vi "Common_UpdateAttributes.vi"(1 "ClassPath/LvClassRef":variant, 2 "NewAttributes":string, 3 "ClassInfo":T4[](array[typedef]), 5 "error in (no error)":errorcluster, 6 "Don't Prompt (False)":bool, 7 "Attributes":T1[](array[typedef]), 8 "Stereotype":string, 9 "Ctl-Description":string) -> (15 "CtlPath":path, 18 "Cancel":bool=TRUE, 19 "error out":errorcluster)   [LabVIEW 2020]
uses:
  <resource>/Framework/Providers/Open_GDS/ClassProviders/Common/CommonVIs/CommonVIs_ClassNamePathType.ctl
  <resource>/Framework/Providers/Open_GDS/ClassProviders/Common/CommonVIs/CommonVIs_AttributeType.ctl
  <resource>/Framework/Providers/Open_GDS/ClassProviders/Common/CommonVIs/CommonVIs_AttributeDataType.ctl
  <resource>/Framework/Providers/Open_GDS/ClassProviders/Common/String/GDSString_AccessScopeModifierType.ctl
  <resource>/Framework/Providers/Open_GDS/ClassProviders/Provider_BaseClassInterface/ClassReader_class/ClassReader.lvclass
panel:
  out "Path":path
  in  "Backup":bool
  out "New Attributes":string
  in  "Cancel":bool
  in  "OK":bool
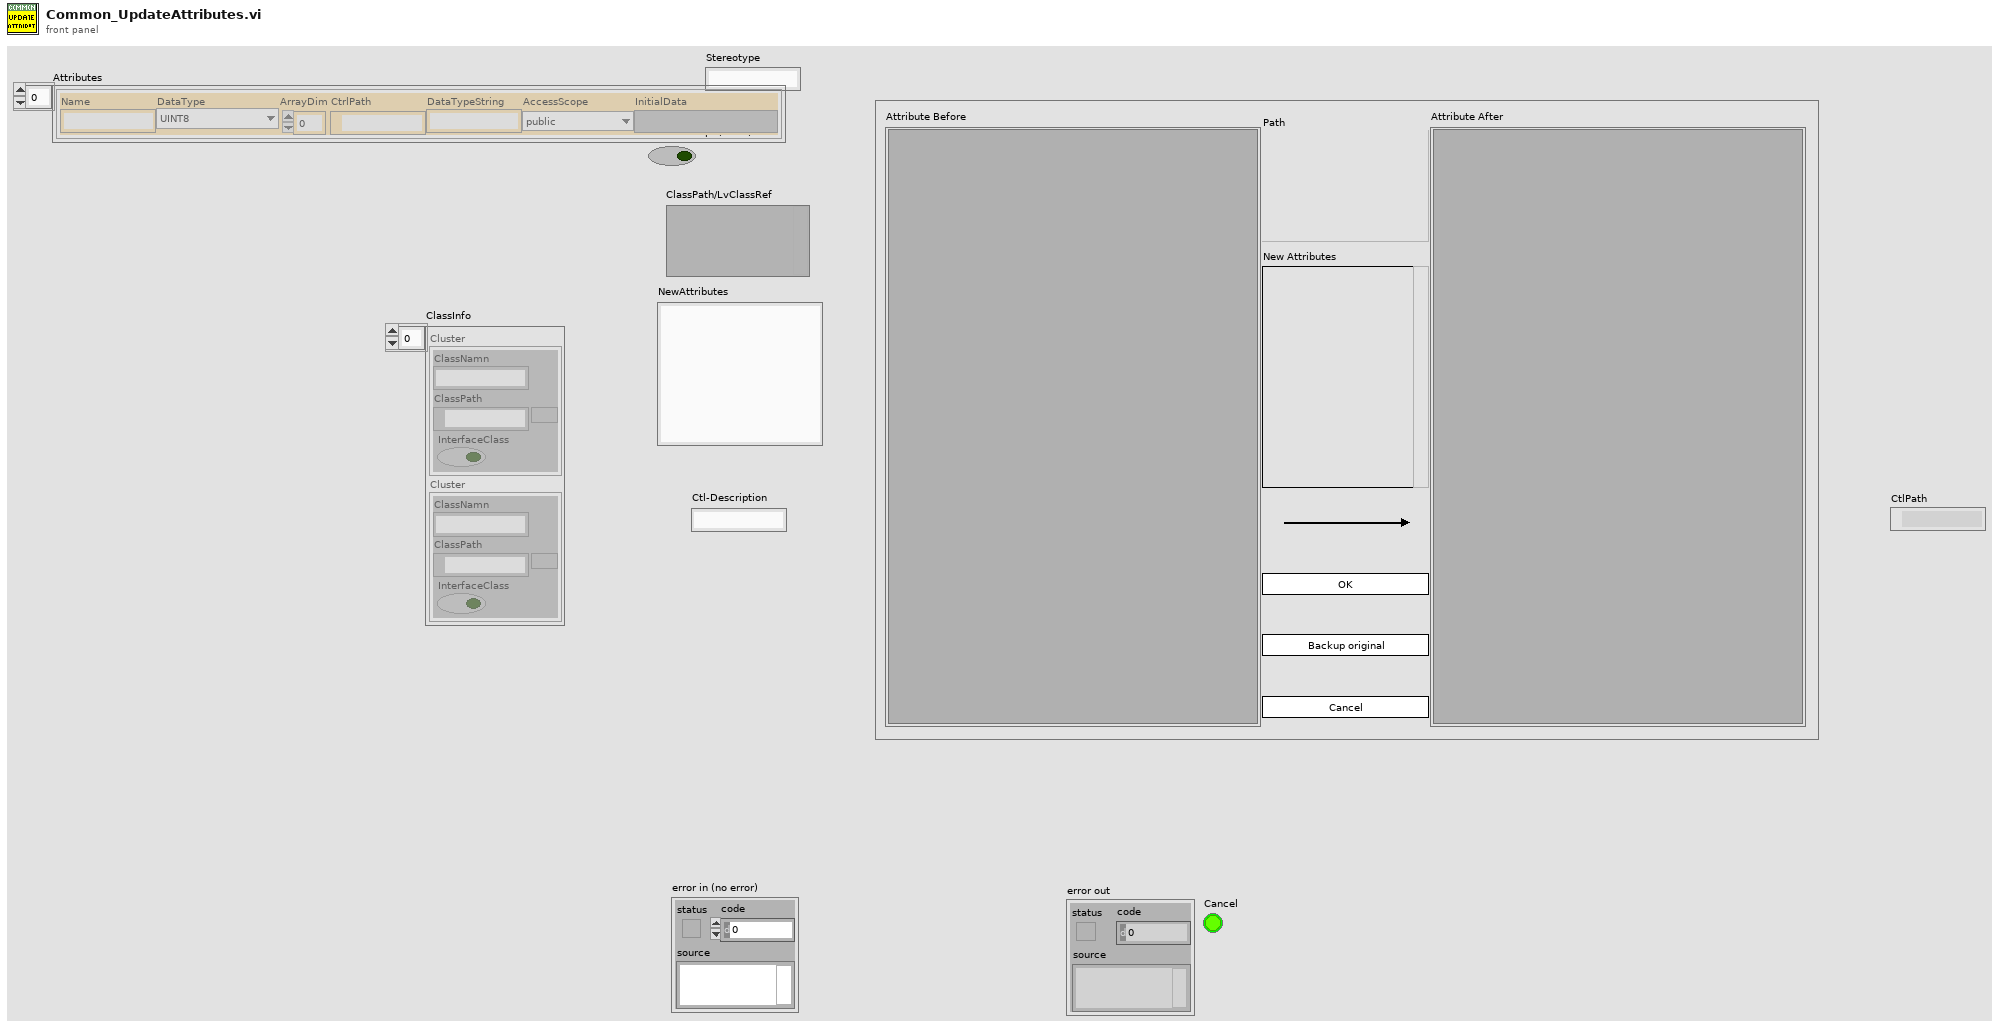
[diagram p1: front panel]
types:
  T1 = typedef "CommonVIs_AttributeType.ctl" = cluster{"Name":string, "DataType":T2, "ArrayDim":i32, "CtrlPath":path, "DataTypeString":string, "AccessScope":T3, "InitialData":variant}
  T2 = typedef "CommonVIs_AttributeDataType.ctl" = enum16{"UINT8", "INT8", "UINT16", "INT16", "UINT32", "INT32", "UINT64", "INT64", "SGL", "DBL", "EXT", "CSG", "CDB", "CXT", "TimeStamp", "STRING", "PATH", "BOOL", "ENUM", "RefNum", "VIRefNum", "LabVIEW Class", "Cluster", "Variant", "TypeDef", "Waveform", "LabVIEW Object", "Other", "void", "Set", "Map"}
  T3 = typedef "GDSString_AccessScopeModifierType.ctl" = enum16{"public", "private", "protected", "internal"}
  T4 = typedef "CommonVIs_ClassNamePathType.ctl" = cluster{"ClassNamn":string, "ClassPath":path, "InterfaceClass":bool}
  T5 = cluster{"OrgCtrl":refnum<vi>, "TemplateControl":path, "NewCtrl":refnum<vi>, "NewCluster":refnum<vi>, "BaseCtrl":refnum<vi>, "AddedCtrls":refnum<vi>[], "Cancel":bool, "Attributes":T1[], "BaseClassType":i16[], "OrgCluster":refnum<vi>, "OrgClusterMembers":cluster{"name":string, "AttributeDataType":T2, "Dims":i16}[], "OrgClusterCtrls":refnum<vi>[], "ClassVi":refnum<vi>, "WaveformControl":path, "EnumControl":path, "Enum":bool, "NewEnum":refnum<vi>, "OrgEnum":refnum<vi>, "ClusterCanBeEmpty":bool, "NewControlCreated":bool, "NoUpdate":bool, "AutoUpdate":bool, "CtlPath":path}
  T6 = enum32{"invalid VI type", "Standard VI", "Control VI", "Global VI", "Polymorphic VI", "Configuration VI"}
  T7 = enum32{"Extended Precision", "Double Precision", "Single Precision", "Long", "Word", "Byte", "Unsigned Long", "Unsigned Word", "Unsigned Byte", "Complex Extended", "Complex Double", "Complex Single", "Quad", "Unsigned Quad"}
  T8 = enum32{"Invalid", "Standard", "Closed", "Hidden", "Minimized", "Maximized"}
  T9 = typedef "CommonVIs_AttributeInfoType.ctl" = cluster{"name":string, "type":T2, "dimension":i32, "typeName":string, "typePath":path, "visibility":T10}
  T10 = typedef "CommonVIs_VisibilityType.ctl" = enum16{"Public", "Private", "Protected"}
  T11 = cluster{"name":string, "AttributeDataType":T2, "Dims":i16}[]
  T12 = cluster{"name":string, "AttributeDataType":T2, "Dims":i16}
  T13 = typedef "LVPointTypeDef.ctl" = cluster{"Horizontal":i16, "Vertical":i16}
  T14 = enum32{"existing file", "new file", "new or existing file", "existing dir", "new dir", "new or existing dir", "existing file (use LLBs)", "new file (use LLBs)", "new or existing file (use LLBs)", "new or existing file or directory (use LLBs)"}
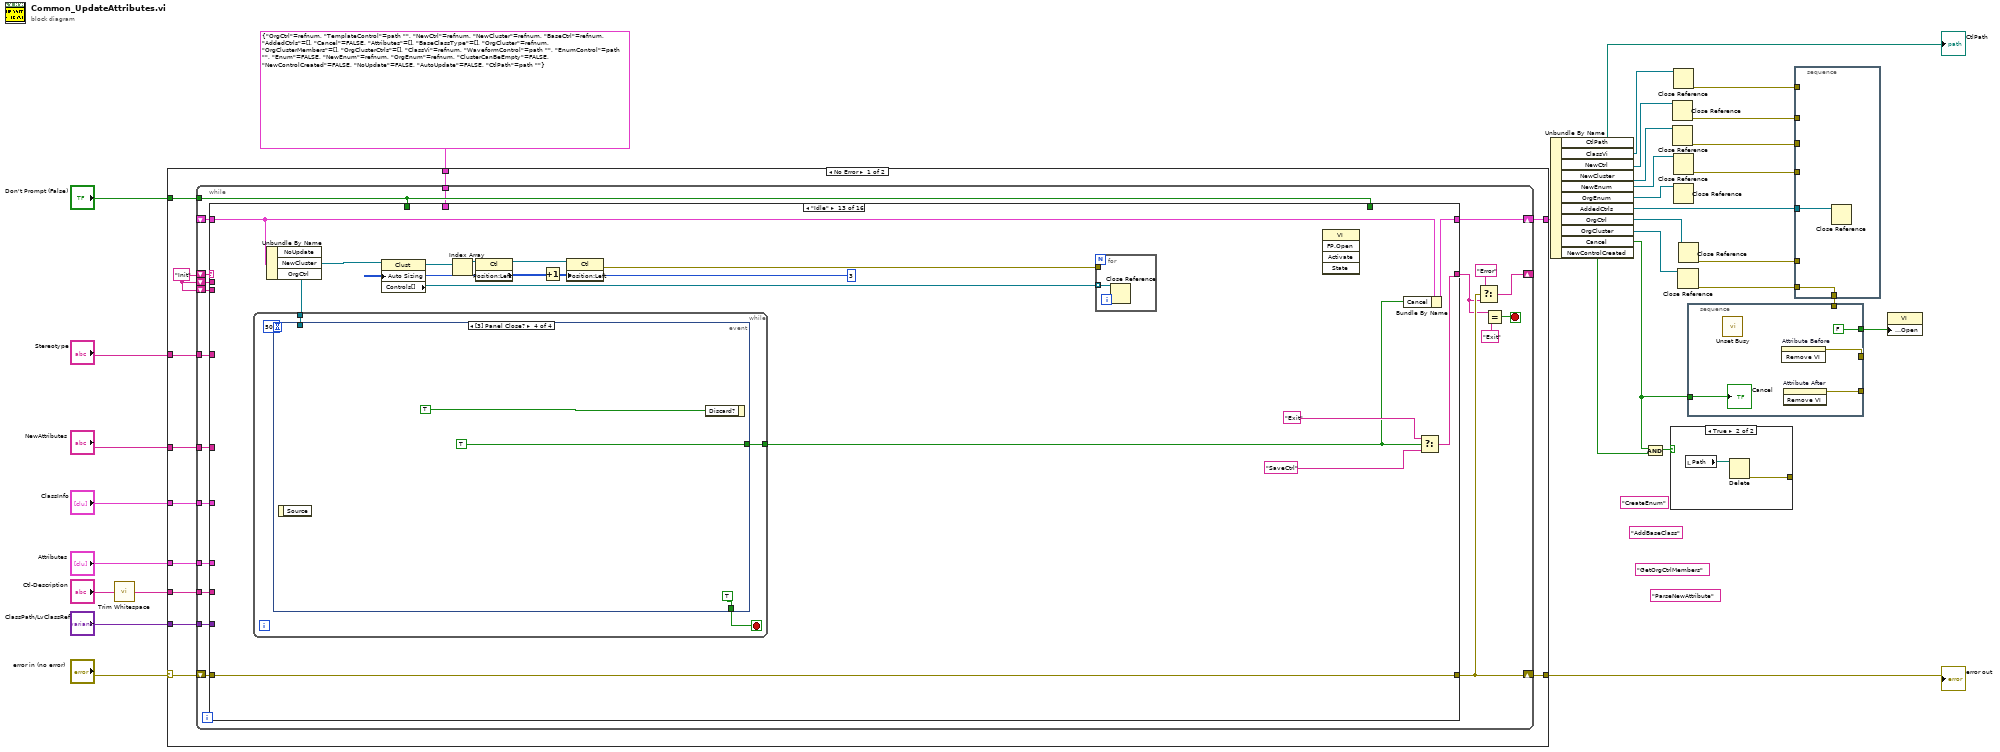
[diagram p0: block diagram]
diagram:
  (unwired) "ParseNewAttribute" ("y")
  (unwired) "GetOrgCtrlMembers" ("y")
  (unwired) "AddBaseClass" ("y")
  (unwired) "CreateEnum" ("y")
  n1 = call <vilib>:"Trim Whitespace.vi"("string"="Ctl-Description") -> ("trimmed string"=w2:string)  [unwired: 1 in]
  n2 = case shown="No Error" "error in (no error)" {
    selector: "error in (no error)" -> [w44 w1117]
    tunnel: [w43 w1117] -> w31
    tunnel: "ClassPath/LvClassRef" -> [w42 _]
    tunnel: [w41 _] -> w22
    tunnel: "NewAttributes" -> [w40 _]
    tunnel: "ClassInfo" -> [w39 _]
    tunnel: "Don't Prompt (False)" -> [w38 _]
    tunnel: "Stereotype" -> [w37 _]
    tunnel: T5 {"OrgCtrl"=refnum, "TemplateControl"=path "", "NewCtrl"=refnum, "NewCluster"=refnum, "BaseCtrl"=refnum, "AddedCtrls"=[], "Cancel"=FALSE, "Attributes"=[], "BaseClassType"=[], "OrgCluster"=refnum, "OrgClusterMembers"=[], "OrgClusterCtrls"=[], "ClassVi"=refnum, "WaveformControl"=path "", "EnumControl"=path "", "Enum"=FALSE, "NewEnum"=refnum, "OrgEnum"=refnum, "ClusterCanBeEmpty"=FALSE, "NewControlCreated"=FALSE, "NoUpdate"=FALSE, "AutoUpdate"=FALSE, "CtlPath"=path ""} -> [w35 _]
    tunnel: "Attributes" -> [w34 _]
    tunnel: w2 -> [w33 _]
    frame No Error {
      w36 = "Init"
      n3 = while {
        shift-right: [w63] -> w43
        shift-left: w44 -> [w64]
        shift-right: [w57] -> _
        shift-left: w36 -> [w62]
        tunnel: w42 -> [w61]
        shift-right: [w60] -> w41
        shift-left: _ -> [w59]
        tunnel: w40 -> [w53]
        tunnel: w39 -> [w52]
        tunnel: w38 -> [w50]
        shift-left: w36 -> [w51]
        tunnel: w37 -> [w49]
        shift-left: w36 -> [w48]
        tunnel: w35 -> [w47]
        tunnel: w34 -> [w46]
        tunnel: w33 -> [w45]
        stop <- w54 stop-if-true
        n4 = case shown="\"Idle\"" w62 {
          tunnel: w64 -> [w72 w130 w208 w268 w302 w364 w392 w428 w453 w474 w506 w857 w877 w940 w1014 w1059]
          tunnel: w61 -> [_ w100 _ _ _ _ _ _ _ _ _ _ _ _ _ _]
          tunnel: [w66 w92 "Init" "AddBaseClass?" w301 "Move Controls" ("y") "GetOrgCtrlMembers" ("y") "ParseNewAttribute" ("y") "None?" ("y") "AddControls" ("y") "Move Controls" ("y") w849 w873 "ReplaceCtrl" ("y") "AddToProject?" ("y") "Exit" ("y")] -> w56
          tunnel: [w70 w128 w202 w259 w298 w359 w381 w425 w450 w466 w503 w845 w872 w935 w949 w1056] -> w60
          tunnel: [w71 w129 w205 w272 w304 w363 w393 w430 w453 w474 w505 w857 w877 w937 w994 w1058] -> w63
          tunnel: w59 -> [w70 _ w202 w262 w293 w359 w382 w423 w451 w464 w491 w845 w870 w935 w981 w1056]
          tunnel: w53 -> [_ w118 _ _ _ w361 _ _ w449 _ _ _ _ _ _ _]
          tunnel: w52 -> [_ _ _ _ _ _ _ _ w439 _ w481 _ _ _ _ _]
          tunnel: w50 -> [_ _ _ _ _ _ _ _ _ _ _ w848 _ _ _ _]
          tunnel: w51 -> [w69 _ _ _ _ _ _ _ _ _ _ _ _ _ _ _]
          tunnel: w50 -> [_ _ _ _ _ _ _ _ _ w465 _ _ _ _ _ _]
          tunnel: w49 -> [_ w107 _ _ _ _ _ _ _ _ _ _ _ _ _ _]
          tunnel: w48 -> [w65 _ _ _ _ _ _ _ _ _ _ _ _ _ _ _]
          tunnel: w47 -> [_ w91 _ _ _ _ _ _ _ _ _ _ _ _ _ _]
          tunnel: w46 -> [_ _ _ _ _ w356 _ _ w442 _ _ _ _ _ _ _]
          tunnel: w45 -> [_ _ _ _ _ _ _ _ _ _ _ _ _ _ w950 _]
          frame "Error", Default {
            n5 = Unbundle By Name(w72) -> ("source"=w68:string, "code"=w67:i32)
            n6 = case shown="0, Default" w67 {
              tunnel: w69 -> [_ w85]
              tunnel: w68 -> [_ _]
              tunnel: w72 -> [w78 _]
              tunnel: [w77 errorcluster {"status"=FALSE, "code"=0, "source"=""}] -> w71
              tunnel: ["Exit" ("y") w87] -> w66
              tunnel: w65 -> [w74 _]
              frame 0, Default {
                n7 = Equal?(x=w74, y="Error" ("t")) -> (x = y?=w73:bool)
                n8 = Select(t=errorcluster {"status"=FALSE, "code"=0, "source"=""}, s=w73, f=w78) -> (s? t:f=w77:errorcluster)
              }
              frame 1073 {
                n9 = call <resource>:"CommonVIs_TwoButtonDialog.vi"("message"="The object attribute file is currently being used by other VIs.\nPlease stop the execution of the VIs that uses this object attributes.", "yesButtonName"="Retry" ("T button name (\"OK\")"), "noButtonName"="Cancel" ("F button name (\"Cancel\")"), "WindowTitle"="Warning") -> ("yesButtonPressed"=w80:bool)  [unwired: 2 in, 13 out]
                n10 = Select(t=w85, s=w80, f="Exit" ("y")) -> (s? t:f=w87:string)
              }
            }
          }
          frame "Init" {
            n11 = Variant To Data(type=path "", Variant=w100) -> (data=w98:path)  [unwired: 1 in, 1 out]
            n12 = Current VI's Path() -> (path=w126:path)
            n13 = call <vilib>:"Get File Extension.vi"("file"=w98) -> ("lowercase file extension"=w99:string)  [unwired: 1 in, 9 out]
            n14 = Strip Path(path=w126) -> (stripped path=w111:path, name=w125:string)
            n15 = case shown="Default" w99 {
              tunnel: w130 -> [w171 w190]
              tunnel: [w171 w189] -> w129
              tunnel: [w169 w173] -> w97
              tunnel: w100 -> [_ w180]
              tunnel: [w170 w172] -> w94
              tunnel: w98 -> [w170 _]
              tunnel: [_ w176] -> w96
              tunnel: [_ w187] -> _
              tunnel: [_ w186] -> _
              frame "ctl" {
                n16 = call <resource>:"CommonVIs_UmlOpenVIRef.vi"("error in"=w171, "ViPath/ViName"=w170) -> ("vi reference"=w169:refnum<vi>)  [unwired: 2 in, 7 out]
              }
              frame Default {
                n17 = call <resource>:"CreateReaderFromClass.vi"("ClassPath/LvClassRef"=w180, "error in"=w190) -> ("ClassReader"=w185:refnum<class "ClassReader.lvclass">, "error out"=w192:errorcluster)  [unwired: 16 out]
                n18 = Variant To Data(type=refnum<vi> refnum ("LVClass.Open"), Variant=w180) -> (error out=w188:errorcluster)  [unwired: 1 in, 1 out]
                n19 = call-dynamic "GetAttributes.vi"("ClassReader in"=w185, "OnlyGetReference"=TRUE, "error in (no error)"=w192) -> ("ClassReader out"=w183:refnum<class "ClassReader.lvclass">, "ObjectAttributeReference"=w174:refnum<vi>, "ClassAttributeReference"=w182:refnum<vi>, "error out"=w191:errorcluster)  [unwired: 13 out]
                n20 = Close Reference(reference=w182) -> (error out=w187:errorcluster)  [unwired: 1 in]
                n21 = case shown="No Error" w188 {
                  tunnel: w183 -> [w193 w196]
                  tunnel: w191 -> [w194 w198]
                  tunnel: [w194 w197] -> w189
                  tunnel: [w193 w195] -> w175
                  frame No Error {
                  }
                  frame Error {
                    n22 = call-dynamic "CleanUp.vi"("reference in"=w196, "error in (no error)"=w198) -> ("reference out"=w195:refnum<class "ClassReader.lvclass">, "error out"=w197:errorcluster)  [unwired: 16 out]
                  }
                }
                n23 = Flatten To String(anything=w175) -> (data string=w177:string)  [unwired: 1 in, 4 out]
                n24 = Match Pattern(string=w177, regular expression="ClassReaderNative") -> (offset past match=w179:i32)  [unwired: 4 out]
                n25 = property class="VI"(reference=w174) -> (reference out=w173:refnum<vi>, error out=w186:errorcluster, "Path"=w172:path)  [unwired: 1 in]
                n26 = Greater Or Equal To 0?(x=w179) -> (x >= 0?=w176:bool)
              }
            }
            "Path" <- w94
            n27 = String Length(string=w125) -> (length=w124:i32)
            n28 = Subtract(x=w124, y=19) -> (x-y=w122:i32)
            n29 = case shown="False" FALSE {
              tunnel: [_ w131] -> w90
              frame False {
              }
              frame True {
                n30 = property class="App"() -> ("App.VersionYear"=w134:string)  [unwired: 2 in, 2 out]
                n31 = Decimal String To Number(string=w134) -> (number=w133:i32)  [unwired: 2 in, 1 out]
                n32 = Greater Or Equal?(x=w133, y=2013) -> (x >= y?=w131:bool)
              }
            }
            n33 = To Upper Case(1:w107) -> (0:w105:string)
            n34 = String Subset(string=w125, offset (0)=0, length (rest)=w122) -> (substring=w113:string)
            n35 = Concatenate Strings(w113, "TemplateObjectAttributes.ctt" ("string")) -> (w120:string)
            n36 = Concatenate Strings(w113, "TemplateWaveform.ctt" ("string")) -> (w114:string)
            n37 = Concatenate Strings(w113, "TemplateEnum.ctt" ("string")) -> (w110:string)
            n38 = Empty String/Path?(string/path=w94) -> (empty?=w93:bool)
            n39 = Build Path(base path=w111, name or relative path=w120) -> (appended path=w109:path)
            n40 = Build Path(base path=w111, name or relative path=w114) -> (appended path=w115:path)
            n41 = Build Path(base path=w111, name or relative path=w110) -> (appended path=w108:path)
            n42 = Match Pattern(string=w105, regular expression="ENUM") -> (offset past match=w104:i32)  [unwired: 4 out]
            n43 = Greater Or Equal To 0?(x=w104) -> (x >= 0?=w103:bool)
            n44 = Select(t=w108, s=w103, f=w109) -> (s? t:f=w102:path)
            n45 = case shown="False" w93 {
              tunnel: [w142 _] -> w127
              tunnel: [w141 _] -> w117
              tunnel: w102 -> [w140 _]
              tunnel: w94 -> [w138 _]
              tunnel: w97 -> [w137 _]
              tunnel: [w136 _] -> w95
              tunnel: ["InsertVI" ("Left Button Text (\"Yes\")") "Exit" ("y")] -> w92
              frame False {
                n46 = Not A Number/Path/Refnum?(number/path/refnum=w137) -> (NaN/Path/Refnum?=w139:bool)
                n47 = case shown="False" w139 {
                  tunnel: [w159 w165] -> w142
                  tunnel: w137 -> [w159 _]
                  tunnel: w140 -> [_ w164]
                  tunnel: [w143 _] -> w141
                  tunnel: w138 -> [w145 w163]
                  tunnel: [_ TRUE] -> w136
                  tunnel: [_ w167] -> _
                  frame False {
                    n48 = Strip Path(path=w145) -> (stripped path=w155:path)  [unwired: 1 out]
                    n49 = Strip Path(path=w155) -> (stripped path=w152:path)  [unwired: 1 out]
                    n50 = List Folder(path=w155, pattern="*Create.vi" ("FileSearchPattern")) -> (filenames=w158:string[])  [unwired: 1 in, 4 out]
                    n51 = List Folder(path=w152, pattern="*Create.vi" ("FileSearchPattern")) -> (path out=w150:path, filenames=w151:string[])  [unwired: 1 in, 3 out]
                    n52 = Array Size(array=w158) -> (size(s)=w157:i32)
                    n53 = Index Array(array=w158) -> (element=w154:string)  [unwired: 1 in]
                    n54 = Index Array(array=w151) -> (element=w149:string)  [unwired: 1 in]
                    n55 = Equal To 0?(x=w157) -> (x = 0?=w148:bool)
                    n56 = Build Path(base path=w155, name or relative path=w154) -> (appended path=w146:path)
                    n57 = Build Path(base path=w150, name or relative path=w149) -> (appended path=w147:path)
                    n58 = Select(t=w147, s=w148, f=w146) -> (s? t:f=w144:path)
                    n59 = call <resource>:"CommonVIs_UmlOpenVIRef.vi"("ViPath/ViName"=w144) -> ("vi reference"=w143:refnum<vi>)  [unwired: 3 in, 7 out]
                  }
                  frame True {
                    # "CREATE FILE"
                    n60 = call <vilib>:"Librarian Copy.vi"("source"=w164, "destination"=w163) -> ("dup destination"=w162:path)  [unwired: 3 in, 6 out]
                    n61 = Set Permissions(7:i16 511 ("permissions"), 11:w162) -> (3:w161:path)  [unwired: 3 in, 1 out]
                    n62 = call <resource>:"CommonVIs_UmlOpenVIRef.vi"("ViPath/ViName"=w161) -> ("error out"=w167:errorcluster, "vi reference"=w165:refnum<vi>)  [unwired: 3 in, 6 out]
                  }
                }
              }
              frame True {
              }
            }
            n63 = Bundle By Name(cluster=w91, "AutoUpdate"=w90, "Enum"=w103, "TemplateControl"=w102, "WaveformControl"=w115, "EnumControl"=w108, "ClusterCanBeEmpty"=w96, "NewControlCreated"=w95, "ClassVi"=w117, "OrgCtrl"=w127) -> (w128:T5)
            "New Attributes" <- w118
          }
          frame "AutoCloseAll" {
            n64 = Unbundle By Name(w202) -> ("OrgCtrl"=w201:refnum<vi>)
            n65 = property class="VI"(reference=w201) -> ("Callers' Names"=w204:string[])  [unwired: 1 in, 2 out]
            n66 = while {
              shift-right: [w218] -> _
              shift-left: w204 -> [w219]
              shift-right: [w222] -> w207
              shift-left: w208 -> [w223]
              shift-right: [w216] -> w200
              shift-left: refnum<vi>[] [] -> [w217]
              stop <- w220 stop-if-true
              n67 = Array Size(array=w219) -> (size(s)=w221:i32)
              n68 = case shown="Default" w221 {
                tunnel: [w227 TRUE] -> w220
                tunnel: w219 -> [w234 w239]
                tunnel: w223 -> [w236 w241]
                tunnel: [w228 w239] -> w218
                tunnel: [w235 w241] -> w222
                tunnel: w217 -> [w226 w238]
                tunnel: [w224 w238] -> w216
                frame Default {
                  n69 = Delete From Array(array=w234, index=0) -> (deleted portion=w232:string, array with subset deleted=w230:string[])  [unwired: 1 in]
                  n70 = Open VI Reference(vi path=w232, error in (no error)=w236) -> (vi reference=w231:refnum<vi>, error out=w237:errorcluster)  [unwired: 4 out]
                  n71 = property class="VI"(reference=w231, error in=w237) -> (reference out=w225:refnum<vi>, error out=w235:errorcluster, "Callers' Names"=w229:string[])
                  n72 = Unbundle By Name(w235) -> ("status"=w227:bool)
                  n73 = Build Array (concatenate)(w230, w229) -> (w228:string[])
                  n74 = Build Array (concatenate)(w226, w225) -> (w224:refnum<vi>[])
                }
                frame 0 {
                }
              }
            }
            n75 = for {
              shift-right: [w214] -> w206
              shift-left: w207 -> [w213]
              tunnel: w200 -> [w209] mode=indexing
              n76 = invoke class="VI" method="Abort VI"(reference=w209, error in=w213) -> (reference out=w211:refnum<vi>)  [unwired: 1 in, 2 out]
              n77 = property class="VI"(reference=w211, error in=w213, "Front Panel Window:Open"=FALSE) -> (reference out=w210:refnum<vi>, error out=w215:errorcluster)
              n78 = Close Reference(reference=w210, error in (no error)=w215) -> (error out=w214:errorcluster)
            }
            n79 = Close Reference(reference=w201, error in (no error)=w206) -> (error out=w205:errorcluster)
          }
          frame "InsertVI" {
            w257 = refnum<vi> refnum  # Enum
            w260 = refnum<vi> refnum  # Cluster
            n80 = Unbundle By Name(w262) -> ("Enum"=w255:bool, "NewControlCreated"=w251:bool, "TemplateControl"=w253:path, "OrgCtrl"=w245:refnum<vi>)
            n81 = call <resource>:"GOOP_AddCtrlToVIIfNeeded.vi"("Ctrl VI in"=w245) -> ("VI out"=w244:refnum<vi>)  [unwired: 8 in, 2 out]
            n82 = invoke class="VI" method="FP.Close"(reference=w244, error in=w268) -> (reference out=w248:refnum<vi>)  [unwired: 1 in, 2 out]
            n83 = invoke on="Attribute Before" class="SubPanel" method="Insert VI"(error in=w268, "VI Ref"=w248) -> (error out=w271:errorcluster)  [unwired: 2 in, 3 out]
            n84 = call <vilib>:"Clear Errors.vi"("error in (no error)"=w271) -> ("error out"=w267:errorcluster)  [unwired: 5 in, 1 out]
            n85 = call <resource>:"CommonVIs_UmlOpenVIRef.vi"("error in"=w267) -> ("error out"=w270:errorcluster, "AppRefOut"=w247:refnum<vi>)  [unwired: 3 in, 6 out]
            n86 = Not A Number/Path/Refnum?(number/path/refnum=w247) -> (NaN/Path/Refnum?=w246:bool)
            n87 = case shown="False" w246 {
              tunnel: T6."Control VI" ("vi type (standard vi)") -> [w281 w287]
              tunnel: [w280 w286] -> w243
              tunnel: w270 -> [w283 w289]
              tunnel: [w282 w288] -> w269
              tunnel: w253 -> [w279 w285]
              tunnel: w247 -> [_ w284]
              frame True {
                n88 = New VI(8:w283, 9:w281, 10:w279) -> (0:w282:errorcluster, 3:w280:refnum<vi>)  [unwired: 4 out]
              }
              frame False {
                n89 = New VI(8:w289, 9:w287, 10:w285, 11:w284) -> (0:w288:errorcluster, 3:w286:refnum<vi>)  [unwired: 3 out]
              }
            }
            n90 = call <resource>:"GOOP_AddCtrlToVIIfNeeded.vi"("Ctrl VI in"=w243) -> ("VI out"=w242:refnum<vi>)  [unwired: 8 in, 2 out]
            n91 = invoke on="Attribute After" class="SubPanel" method="Insert VI"(error in=w269, "VI Ref"=w242) -> (error out=w278:errorcluster)  [unwired: 2 in, 3 out]
            n92 = call <vilib>:"Clear Errors.vi"("error in (no error)"=w278) -> ("error out"=w266:errorcluster)  [unwired: 5 in, 1 out]
            n93 = property class="VI"(reference=w242, error in=w266) -> (error out=w276:errorcluster, "Front Panel"=w264:refnum<vi>)  [unwired: 1 out]
            n94 = property class="Pnl"(reference=w264, error in=w276) -> (reference out=w261:refnum<vi>, error out=w277:errorcluster, "Controls[]"=w263:refnum<vi>[])
            n95 = local read "Path"() -> (w250:path)
            n96 = Index Array(array=w263) -> (element=w256:refnum<vi>)  [unwired: 1 in]
            n97 = call <vilib>:"Get File Extension.vi"("file"=w250) -> ("filename without extension"=w249:string)  [unwired: 1 in, 9 out]
            n98 = Close Reference(reference=w261, error in (no error)=w277) -> (error out=w275:errorcluster)
            n99 = To More Specific Class(target class=w257, reference=w256, error in=w275) -> (specific class reference=w254:refnum<vi>, error out=w274:errorcluster)
            n100 = To More Specific Class(target class=w260, reference=w256, error in=w275) -> (specific class reference=w252:refnum<vi>, error out=w273:errorcluster)
            n101 = Select(t=w274, s=w255, f=w273) -> (s? t:f=w272:errorcluster)
            n102 = Bundle By Name(cluster=w262, "NewCtrl"=w242, "NewEnum"=w254, "NewCluster"=w252) -> (w259:T5)
            n103 = case shown="False" w251 {
              tunnel: w252 -> [_ w291]
              tunnel: w249 -> [_ w290]
              frame False {
              }
              frame True {
                n104 = property class="Clust"(reference=w291, "Label.Text"=w290) -> ()  [unwired: 1 in, 2 out]
              }
            }
          }
          frame "AddBaseClass?" {
            w300 = refnum<vi> refnum  # Cluster
            n105 = Unbundle By Name(w293) -> ("Enum"=w292:bool)
            n106 = Unbundle By Name(w293) -> ("OrgCtrl"=w296:refnum<vi>)
            n107 = property class="VI"(reference=w296, error in=w302) -> (error out=w306:errorcluster, "Front Panel"=w295:refnum<vi>)  [unwired: 1 out]
            n108 = property class="Pnl"(reference=w295, error in=w306) -> (error out=w305:errorcluster, "Controls[]"=w299:refnum<vi>[])  [unwired: 1 out]
            n109 = Index Array(array=w299) -> (element=w294:refnum<vi>)  [unwired: 1 in]
            n110 = To More Specific Class(target class=w300, reference=w294, error in=w305) -> (specific class reference=w297:refnum<vi>, error out=w303:errorcluster)
            n111 = case shown="No Error" w303 {
              tunnel: [w309 w343] -> w301
              tunnel: w303 -> [w320 _]
              tunnel: w293 -> [w317 w340]
              tunnel: [w316 w339] -> w298
              tunnel: [w322 w345] -> w304
              tunnel: w297 -> [w314 _]
              tunnel: w302 -> [_ w345]
              tunnel: w294 -> [_ w342]
              tunnel: w292 -> [w307 w337]
              frame No Error {
                # "Base Class Type"
                # "BaseClass Found"
                n112 = property class="Clust"(reference=w314, error in=w320) -> (error out=w321:errorcluster, "Controls[]"=w312:refnum<vi>[])  [unwired: 1 out]
                n113 = for {
                  N: 1 -> [_]
                  tunnel: w320 -> [w333]
                  tunnel: [w327] -> w311
                  tunnel: [w325] -> w315
                  tunnel: w312 -> [w323] mode=indexing
                  w324 = "Base class" ("x")
                  n114 = property class="Ctl"(reference=w323, error in=w333) -> ("Label.Text"=w330:string, "Class Name"=w332:string, "Type Descriptor"=w326:i16[])  [unwired: 2 out]
                  n115 = Equal?(x=w332, y="Cluster") -> (x = y?=w328:bool)
                  n116 = Equal?(x=w324, y=w330) -> (x = y?=w329:bool)
                  n117 = And(x=w329, y=w328) -> (x .and. y?=w327:bool)
                  n118 = call <resource>:"CommonVIs_TypeDescNonNameDepentent.vi"("Type DescriptorNameDependent"=w326, "LabelText"=w324) -> ("Type DescriptorNonNameDependent"=w325:i16[])  [unwired: 17 out]
                }
                n119 = for {
                  shift-right: [w335] -> w322
                  shift-left: w321 -> [w336]
                  tunnel: w312 -> [w334] mode=indexing
                  tunnel: w311 -> [_]
                  n120 = Close Reference(reference=w334, error in (no error)=w336) -> (error out=w335:errorcluster)
                }
                n121 = Bundle By Name(cluster=w317, "OrgCluster"=w314, "BaseClassType"=w315) -> (w316:T5)
                n122 = Select(t="AddBaseClass" ("y"), s=w311, f="GetOrgCtrlMembers" ("y")) -> (s? t:f=w310:string)
                n123 = Select(t="CreateEnum" ("y"), s=w307, f=w310) -> (s? t:f=w309:string)
              }
              frame Error {
                w341 = refnum<vi> refnum  # Enum
                n124 = To More Specific Class(target class=w341, reference=w342) -> (specific class reference=w338:refnum<vi>, error out=w344:errorcluster)  [unwired: 1 in]
                n125 = case shown="No Error" w344 {
                  tunnel: [w347 "Exit" ("y")] -> w343
                  tunnel: w340 -> [w352 w353]
                  tunnel: [w351 w353] -> w339
                  tunnel: w338 -> [w350 _]
                  tunnel: w337 -> [w349 _]
                  frame No Error {
                    n126 = Select(t="CreateEnum" ("y"), s=w349, f="ParseNewAttribute" ("y")) -> (s? t:f=w347:string)
                    n127 = Bundle By Name(cluster=w352, "OrgEnum"=w350) -> (w351:T5)
                  }
                  frame Error {
                    n128 = One Button Dialog(message="Only cluster controls are supported") -> ()  [unwired: 2 out]
                  }
                }
              }
            }
          }
          frame "CreateEnum" {
            n129 = Empty Array?(array=w356) -> (empty?=w357:bool)
            n130 = Unbundle By Name(w359) -> ("NewEnum"=w362:refnum<vi>)
            n131 = case shown="False" w357 {
              tunnel: w361 -> [_ w374]
              tunnel: [w365 w369] -> w360
              tunnel: w356 -> [w366 _]
              frame False {
                n132 = for {
                  tunnel: w366 -> [w368] mode=indexing
                  tunnel: [w367] -> w365 mode=indexing
                  n133 = Unbundle By Name(w368) -> ("Name"=w367:string)
                }
              }
              frame True {
                n134 = call <vilib>:"Trim Whitespace.vi"("string"=w374) -> ("trimmed string"=w373:string)  [unwired: 1 in]
                n135 = Spreadsheet String To Array(delimiter (Tab)="\n", format string="%s", spreadsheet string=w373, array type (2D Dbl)=string[] []) -> (array=w369:string[])
              }
            }
            n136 = property class="Enum"(reference=w362, error in=w364, "Strings []"=w360) -> (error out=w363:errorcluster)  [unwired: 1 out]
          }
          frame "AddBaseClass" {
            w387 = refnum<vi> refnum  # Cluster
